vi "Drive for Time.vi"(7 "Description":string, 8 "Command Info In":T1, 10 "Duration":dbl, 11 "Speed (-1 to 1)":dbl) -> (0 "Command Info Out":T1)   [LabVIEW 2015]
uses:
  <vilib>/Rock Robotics/WPI/Framework/Command Status Info.ctl
  <vilib>/Rock Robotics/WPI/Framework/Completion Status.ctl
  <vilib>/Rock Robotics/WPI/Framework/Completion Notifier.ctl
  Implementation/Drive Setpoints.ctl
  Implementation/Drive Operations.ctl
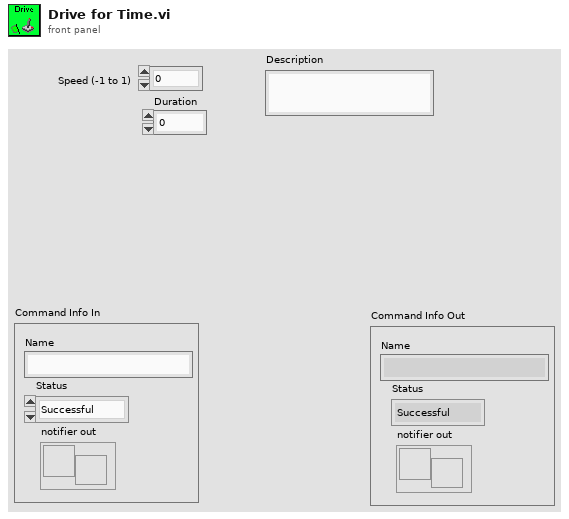
[diagram p1: front panel]
types:
  T1 = typedef "Command Status Info.ctl" = cluster{"Name":string, "Status":T2, "notifier out":T3}
  T2 = typedef "Completion Status.ctl" = enum16{"Successful", "Aborted", "Incomplete"}
  T3 = typedef "Completion Notifier.ctl" = refnum<notifier>
  T4 = typedef "Drive Setpoints.ctl" = cluster{"Operation":T5, "Left Setpoint":dbl, "Duration":dbl, "Right Setpoint":dbl}
  T5 = typedef "Drive Operations.ctl" = enum16{"Reserve", "Read Current", "Immediate", "Turn to Angle", "Drive for Distance", "Drive for Time"}
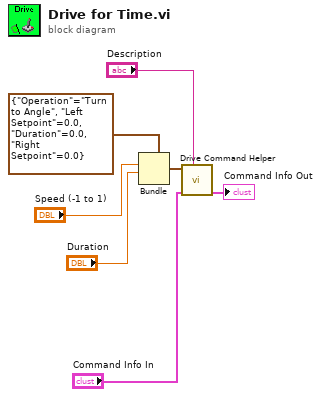
[diagram p0: block diagram]
diagram:
  n1 = Bundle(cluster=T4 {"Operation"=enum."Turn to Angle", "Left Setpoint"=0.0, "Duration"=0.0, "Right Setpoint"=0.0} ("SubSystem Data"), "Left Setpoint"="Speed (-1 to 1)", "Duration"="Duration") -> (w2:T4)  [unwired: 2 in]
  n2 = call "Drive Command Helper.vi"("Description"="Description", "Command Info In"="Command Info In", "SubSystem Data"=w2) -> ("Command Info Out"=→"Command Info Out":T1)  [unwired: 7 in, 1 out]
